vi "NIDCPower_channel_ganging - export signal.vi"(7 "signal identifier (none)":string, 8 "error in (no error)":errorcluster, 9 "output terminal":tag, 10 "signal":T1=1030 items=["Source Complete Event"=1030, "Measure Complete Event"=1031, "Sequence Iteration Complete Event"=1032, "Sequence Engine Done Event"=1033, "Pulse Complete Event"=1051, "Ready For Pulse Trigger Event"=1052, "Start Trigger"=1034, "Source Trigger"=1035, "Measure Trigger"=1036, "Sequence Advance Trigger"=1037, "Pulse Trigger"=1053], 11 "Ganged Session in":T2) -> (0 "error out":errorcluster, 3 "Ganged Session out":T2)   [LabVIEW 2021]
uses:
  ctl/NIDCPower_channel_ganging - ctl - ganged session.ctl
  ctl/NIDCPower_channel_ganging - ctl - ganged config.ctl
  ctl/NIDCPower_channel_ganging - ctl - channel mode.ctl
  <instrlib>/niDCPower/nidcpower.llb/niDCPower Export Signal - Signal.ctl
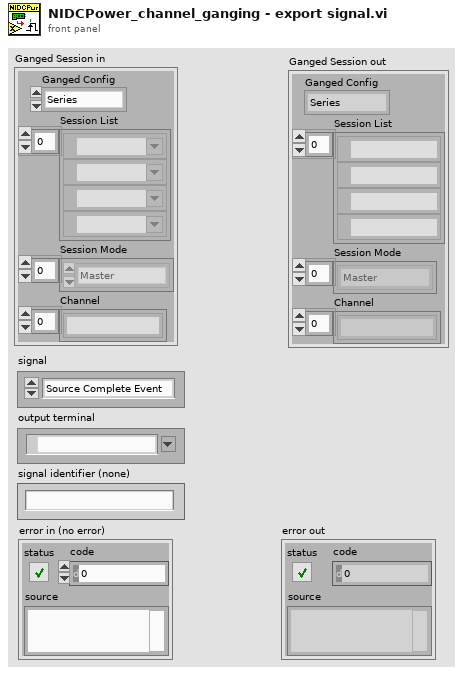
[diagram p1: front panel]
types:
  T1 = typedef "niDCPower Export Signal - Signal.ctl" = i32
  T2 = typedef "NIDCPower_channel_ganging - ctl - ganged session.ctl" = cluster{"Ganged Config":T3, "Session List":refnum<k15>[], "Session Mode":T4[], "Channel":string[]}
  T3 = typedef "NIDCPower_channel_ganging - ctl - ganged config.ctl" = enum32{"Series", "Parallel", "Manual"}
  T4 = typedef "NIDCPower_channel_ganging - ctl - channel mode.ctl" = enum32{"Master", "Slave", "Slave - Inverted"}
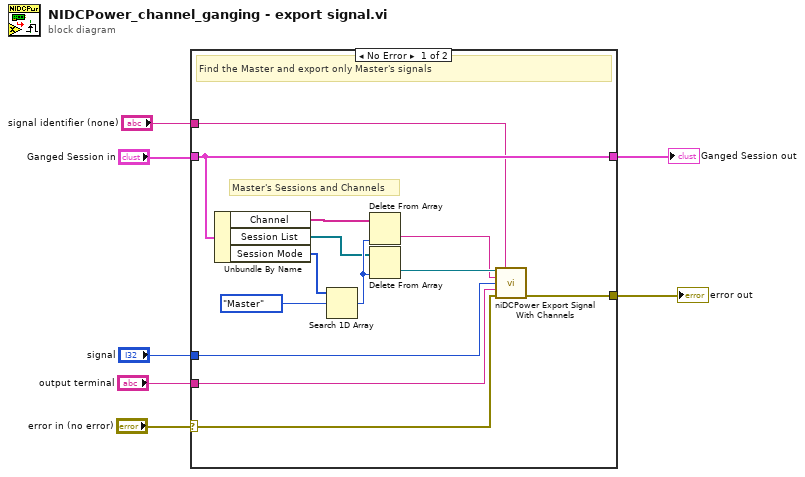
[diagram p0: block diagram]
diagram:
  n1 = case shown="No Error" "error in (no error)" {
    selector: "error in (no error)" -> [w13 w22]
    tunnel: [w9 w22] -> w7
    tunnel: "Ganged Session in" -> [w19 w21]
    tunnel: [w19 w21] -> w5
    tunnel: "signal" -> [w12 _]
    tunnel: "output terminal" -> [w11 _]
    tunnel: "signal identifier (none)" -> [w8 _]
    frame No Error {
      # "Master's Sessions and Channels"
      # "Find the Master and export only Master's signals"
      n2 = Unbundle By Name(w19) -> ("Channel"=w17:string[], "Session List"=w16:refnum<k15>[], "Session Mode"=w15:T4[])
      n3 = Search 1D Array(1D array=w15, element=NIDCPower_channel_ganging_-_ctl_-_channel_mode."Master" ("Channel Mode")) -> (index of element=w18:i32)  [unwired: 1 in]
      n4 = Delete From Array(array=w17, index=w18) -> (deleted portion=w10:string)  [unwired: 1 in, 1 out]
      n5 = Delete From Array(array=w16, index=w18) -> (deleted portion=w14:refnum<k15>)  [unwired: 1 in, 1 out]
      n6 = call <instrlib>:"niDCPower Export Signal With Channels.vi"("instrument handle"=w14, "signal identifier (none)"=w8, "channel name"=w10, "signal"=w12, "output terminal"=w11, "error in (no error)"=w13) -> ("error out"=w9:errorcluster)  [unwired: 8 in, 1 out]
    }
    frame Error {
    }
  }
  "error out" <- w7
  "Ganged Session out" <- w5
